vi "Replace Node.vi"(7 "Children In Place? (F)":bool, 8 "error in (no error)":errorcluster, 9 "New Node":refnum<data-value>, 10 "Old Node":refnum<data-value>, 11 "AST in":refnum<class "AST.lvclass">) -> (0 "error out":errorcluster, 3 "AST out":refnum<class "AST.lvclass">)   [LabVIEW 2020, in "PicoG-ParserLexer.lvlib" / "AST.lvclass"]
uses:
  AST.lvclass
  Node/Node.lvclass
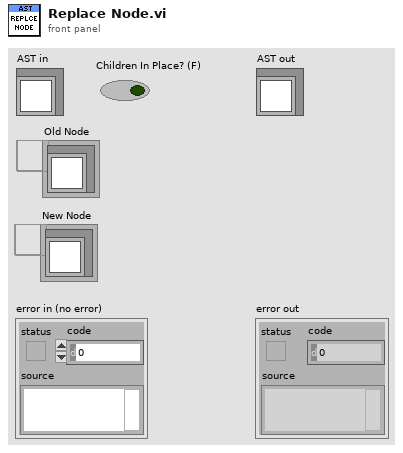
[diagram p1: front panel]
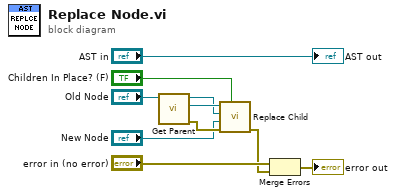
[diagram p0: block diagram]
diagram:
  n1 = call "Get Parent.vi"("NodeRef In"="Old Node") -> ("error out"=w10:errorcluster, "Parent"=w5:refnum<data-value>, "NodeRef"=w4:refnum<data-value>)  [unwired: 8 in]
  n2 = call "Replace Child.vi"("Children In Place? (F)"="Children In Place? (F)", "error in (no error)"=w10, "New Node"="New Node", "Old Node"=w4, "NodeRef In"=w5) -> ("error out"=w1:errorcluster)  [unwired: 5 in, 1 out]
  n3 = Merge Errors("error in (no error)", w1) -> (→"error out":errorcluster)
  "AST out" <- "AST in"
